vi "Read Services.vi"(8 "error in (no error)":errorcluster, 11 "CS++DIMMonitor in":refnum<class "CS++DIMMonitor.lvclass">) -> (0 "error out":errorcluster, 2 "Services":string[](array[string]), 3 "CS++DIMMonitor out":refnum<class "CS++DIMMonitor.lvclass">)   [LabVIEW 2015, in "CS++DIMMonitor.lvlib" / "CS++DIMMonitor.lvclass"]
doc: "Read Services from attribute."
uses:
  CS++DIMMonitor.lvclass
  CS++DIMMonitor.lvclass/CS++DIMMonitor.ctl
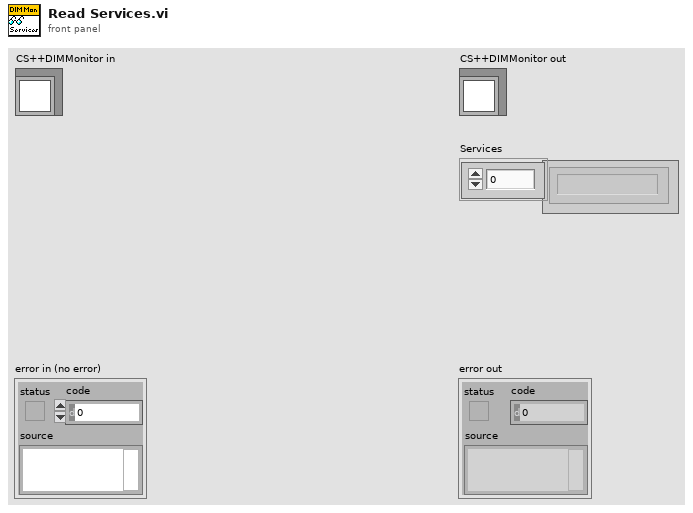
[diagram p1: front panel]
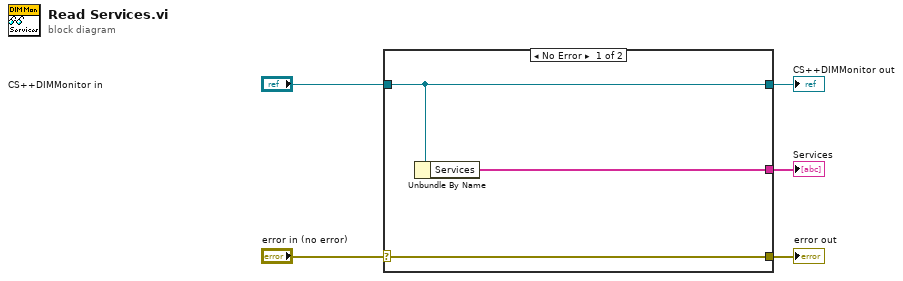
[diagram p0: block diagram]
diagram:
  n1 = case shown="No Error" "error in (no error)" {
    selector: "error in (no error)" -> [w8 w9]
    tunnel: [w8 w9] -> w4
    tunnel: [w7 w10] -> w2
    tunnel: "CS++DIMMonitor in" -> [w7 w10]
    tunnel: [w6 _] -> w1
    frame No Error {
      n2 = Unbundle By Name(w7) -> ("Services"=w6:string[])
    }
    frame Error {
    }
  }
  "error out" <- w4
  "CS++DIMMonitor out" <- w2
  "Services" <- w1
